vi "CamServer global.vi"() -> ()   [LabVIEW 2020]
uses:
  Camera enum/Camera enum.ctl
panel:
  out "Image Pathnames":path[](array[path])
  in  "Image Saved?":refnum<k4>
  in  "Demanded Local cameras":T1[](array[typedef])=["Travcam", "Tunnelcam", "Pencilcam"]
  in  "CamServer machine name or IP":string="EnFlo-CamServer"
  in  "Scratch file directory":path=path "\\\\EnFlo-Data\\Public/CamServer"
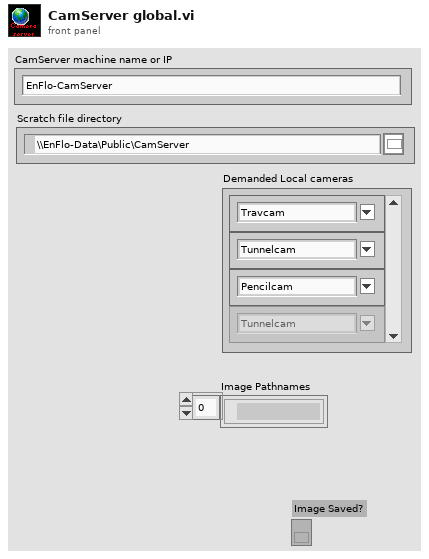
[diagram p1: front panel]
types:
  T1 = typedef "Camera enum.ctl" = string
diagram:
